vi "Wait for UDP connection.vi"(8 "error in (no error)":errorcluster, 9 "Timeout (-1 never timeout)":i32=-1, 10 "port (60200)":u16=60200) -> (0 "error out":errorcluster, 2 "Initial teleop command":T1, 3 "UDP Network Connection out":refnum<k16>)   [LabVIEW 2012]
doc: "Waits for a UDP message on the specified port that matches the teleop command datatype."
uses:
  Teleop command.ctl
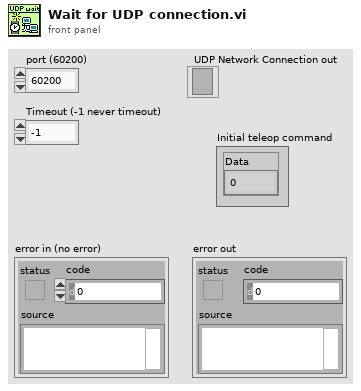
[diagram p1: front panel]
types:
  T1 = typedef "Teleop command.ctl" = cluster{"Data":dbl}
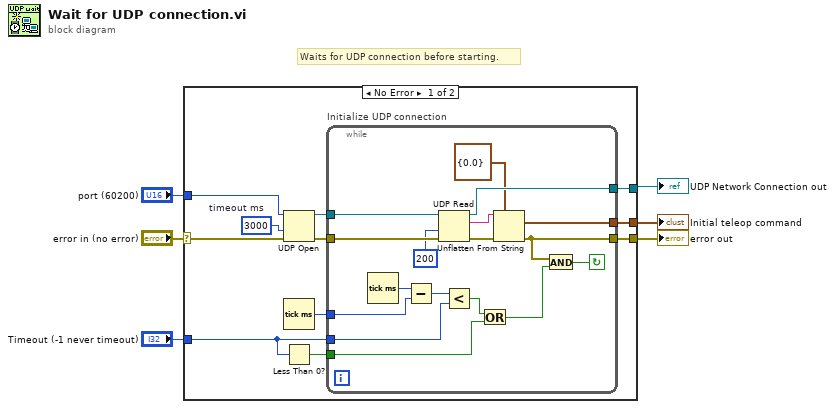
[diagram p0: block diagram]
diagram:
  # "Waits for UDP connection before starting."
  n1 = case shown="No Error" "error in (no error)" {
    selector: "error in (no error)" -> [w10 w35]
    tunnel: [w17 _] -> w1
    tunnel: [w16 w35] -> w6
    tunnel: [w15 _] -> w5
    tunnel: "port (60200)" -> [w12 _]
    tunnel: "Timeout (-1 never timeout)" -> [w8 _]
    frame No Error {
      w11 = 3000  # timeout ms
      n2 = UDP Open(8:w10, 9:w11, 11:w12) -> (port=w13:refnum<k16>, 0:w14:errorcluster)  [unwired: 2 in, 1 out]
      n3 = Tick Count (ms)() -> (millisecond timer value=w9:u32)
      n4 = Less Than 0?(x=w8) -> (x < 0?=w7:bool)
      n5 = while "Initialize UDP connection" {
        tunnel: w13 -> [w34]
        tunnel: [w33] -> w15
        tunnel: w14 -> [w32]
        tunnel: [w24] -> w16
        tunnel: [w29] -> w17
        tunnel: w9 -> [w27]
        tunnel: w8 -> [w25]
        tunnel: w7 -> [w21]
        stop <- w23 continue-if-true
        n6 = Tick Count (ms)() -> (millisecond timer value=w28:u32)
        n7 = Subtract(x=w28, y=w27) -> (x-y=w26:u32)
        n8 = UDP Read(connection ID=w34, timeout ms (25000)=200, 8:w32) -> (data out=w31:string, error out=w30:errorcluster, 3:w33:refnum<k16>)  [unwired: 1 in, 2 out]
        n9 = Less?(x=w26, y=w25) -> (x < y?=w22:bool)
        n10 = Or(x=w22, y=w21) -> (x .or. y?=w20:bool)
        n11 = Unflatten From String(type=T1 {"Data"=0.0} ("Teleop command"), binary string=w31, error in (no error)=w30) -> (value=w29:T1, error out=w24:errorcluster)  [unwired: 2 in, 1 out]
        n12 = And(x=w24, y=w20) -> (x .and. y?=w23:bool)
      }
    }
    frame Error {
    }
  }
  "error out" <- w6
  "UDP Network Connection out" <- w5
  "Initial teleop command" <- w1
